vi "Steering Encoder Counter.vi"   [LabVIEW 2009]
uses:
  Motor Control Global.vi
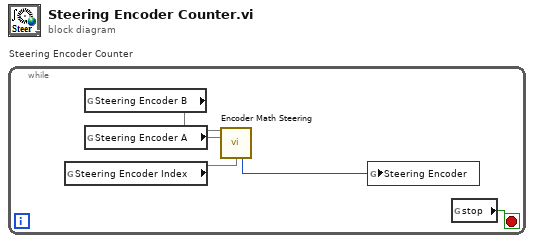
[diagram p0: block diagram]
diagram:
  n1 = while "Steering Encoder Counter" {
    stop <- w5 stop-if-true
    n2 = global read "Motor Control Global.vi" "Steering Encoder Index"() -> (w2)
    n3 = global read "Motor Control Global.vi" "Steering Encoder B"() -> (w4)
    n4 = global read "Motor Control Global.vi" "Steering Encoder A"() -> (w3)
    n5 = call "Encoder Math Steering.vi"("Encoder B"=w4, "Encoder A"=w3, "Encoder Index"=w2) -> ("Current count"=w1:i32)  [unwired: 9 in, 3 out]
    n6 = global write "Motor Control Global.vi" "Steering Encoder"(w1) -> ()
    n7 = global read "Motor Control Global.vi" "stop"() -> (w5:bool)
  }
